vi "MB MFC Setpoint+.vi"(7 "Action":T1, 8 "error in (no error)":errorcluster, 9 "Setpoint":sgl, 11 "TCP Ref":refnum<k5>) -> (0 "error out":errorcluster, 1 "Setpoint":sgl, 3 "dup TCP Ref":refnum<k5>)   [LabVIEW 2011]
doc: "This VI reads or writes the setpoint of an MKS Modbus MFC. If this VI is told to write a setpoint, it will write it and then read it to make sure that the desired setpoint was set."
uses:
  Type Definitions/Modbus Action.ctl
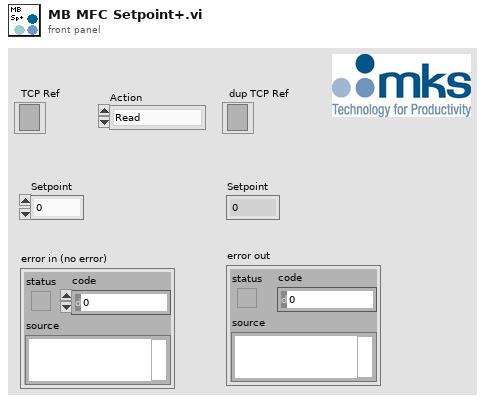
[diagram p1: front panel]
types:
  T1 = typedef "Modbus Action.ctl" = enum16{"Read", "Write"}
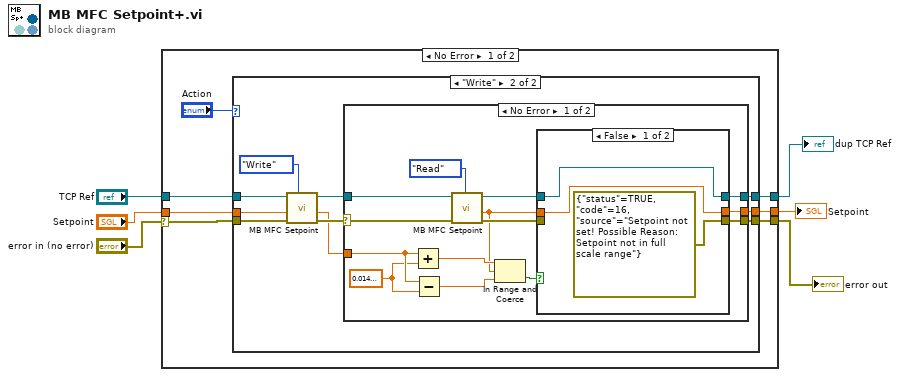
[diagram p0: block diagram]
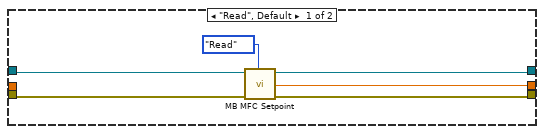
[diagram p2: hidden frame]
diagram:
  n1 = case shown="No Error" "error in (no error)" {
    selector: "error in (no error)" -> [w11 w53]
    tunnel: "TCP Ref" -> [w13 w55]
    tunnel: "Setpoint" -> [w12 w54]
    tunnel: [w10 w55] -> w3
    tunnel: [w9 w53] -> w2
    tunnel: [w8 w54] -> w1
    frame No Error {
      n2 = case shown="\"Write\"" "Action" {
        tunnel: w13 -> [w14 w29]
        tunnel: w12 -> [_ w28]
        tunnel: w11 -> [w18 w25]
        tunnel: [w15 w22] -> w10
        tunnel: [w17 w21] -> w9
        tunnel: [w16 w20] -> w8
        frame "Read", Default {
          n3 = call "MB MFC Setpoint.vi"("Action"=Modbus_Action."Read", "error in (no error)"=w18, "TCP Ref"=w14) -> ("error out"=w17:errorcluster, "Setpoint"=w16:sgl, "dup TCP Ref"=w15:refnum<k5>)  [unwired: 6 in]
        }
        frame "Write" {
          n4 = call "MB MFC Setpoint.vi"("Action"=Modbus_Action."Write", "error in (no error)"=w25, "Setpoint"=w28, "TCP Ref"=w29) -> ("error out"=w24:errorcluster, "Setpoint"=w23:sgl, "dup TCP Ref"=w27:refnum<k5>)  [unwired: 5 in]
          n5 = case shown="No Error" w24 {
            selector: w24 -> [w41 w51]
            tunnel: w27 -> [w43 w50]
            tunnel: w23 -> [w40 w52]
            tunnel: [w34 w50] -> w22
            tunnel: [w33 w51] -> w21
            tunnel: [w31 w52] -> w20
            frame No Error {
              w39 = sgl 0.015 ("y")
              n6 = Add(x=w40, y=w39) -> (x+y=w38:sgl)
              n7 = Subtract(x=w40, y=w39) -> (x-y=w37:sgl)
              n8 = call "MB MFC Setpoint.vi"("Action"=Modbus_Action."Read", "error in (no error)"=w41, "TCP Ref"=w43) -> ("error out"=w32:errorcluster, "Setpoint"=w30:sgl, "dup TCP Ref"=w35:refnum<k5>)  [unwired: 6 in]
              n9 = In Range and Coerce(upper limit=w38, x=w30, lower limit=w37) -> (In Range?=w36:bool)  [unwired: 1 out]
              n10 = case shown="False" w36 {
                tunnel: [w45 w49] -> w34
                tunnel: w35 -> [w45 w49]
                tunnel: [errorcluster {"status"=TRUE, "code"=16, "source"="Setpoint not set! Possible Reason: Setpoint not in full scale range"} ("error out") w48] -> w33
                tunnel: w32 -> [_ w48]
                tunnel: [w44 w47] -> w31
                tunnel: w30 -> [w44 w47]
                frame False {
                }
                frame True {
                }
              }
            }
            frame Error {
            }
          }
        }
      }
    }
    frame Error {
    }
  }
  "Setpoint" <- w1
  "dup TCP Ref" <- w3
  "error out" <- w2
